vi "proba_kor_xy.vi"() -> ()   [LabVIEW 2012]
panel:
  out "XY Graph 2":cluster{"X":dbl[], "Y":dbl[]}[](graph)
  in  "Size":dbl(slide)=0.19732441471571907 scale=0.0..1.0
  in  "stop":bool
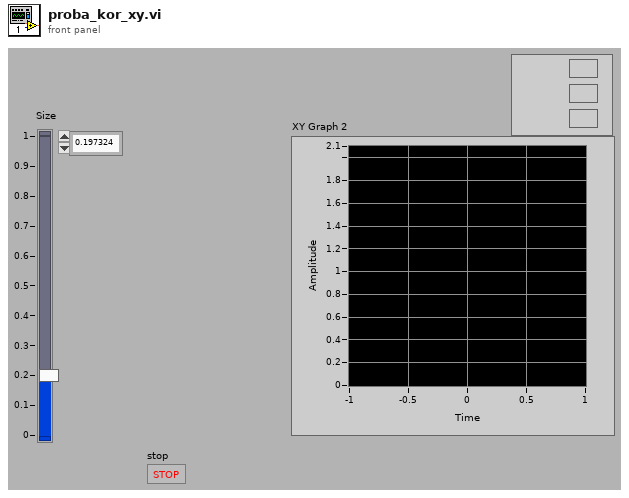
[diagram p1: front panel]
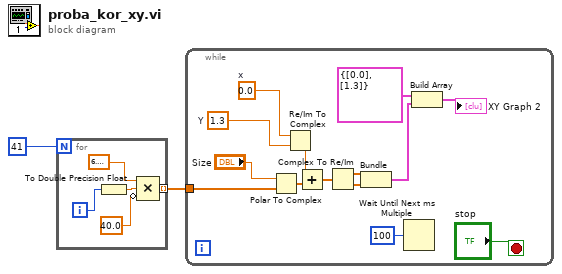
[diagram p0: block diagram]
diagram:
  n1 = for {
    N: 41 -> [_]
    tunnel: [w3] -> w1 mode=indexing
    i -> [w7]
    n2 = To Double Precision Float(number=w7) -> (double precision float=w4:dbl)
    n3 = Compound Arithmetic op=MULTIPLY(6.283185307179586, w4, invert 40.0 ("value")) -> (w3:dbl)
  }
  n4 = while {
    tunnel: w1 -> [w12]
    stop <- "stop" stop-if-true
    w18 = 1.3  # Y
    w19 = 0.0  # x
    n5 = Polar To Complex(1:w12, 2:"Size") -> (0:w11:cdb[])
    n6 = Re/Im To Complex(1:w18, 2:w19) -> (0:w17:cdb)
    n7 = Add(x=w17, y=w11) -> (x+y=w16:cdb[])
    n8 = Complex To Re/Im(x + iy=w16) -> (x=w15:dbl[], y=w14:dbl[])
    n9 = Bundle(w15, w14) -> (w10:cluster{dbl[], dbl[]})  [unwired: 1 in]
    n10 = Wait Until Next ms Multiple(millisecond multiple=u32 100) -> ()  [unwired: 1 out]
    n11 = Build Array(cluster{dbl[], dbl[]} {[0.0], [1.3]} ("element"), w10) -> (→"XY Graph 2":cluster{dbl[], dbl[]}[])
  }
